vi "UDP LA SEND.vi"() -> ()   [LabVIEW 2017]
uses:
  Global 1.vi
panel:
  in  "upper limit":dbl
  in  "lower limit":dbl
  in  "*/":dbl
  in  "+-":i32
  in  "*/compensate":bool
  in  "+-compensate":bool
  out "LA position":i32
  out "decimal integer string":string
  in  "number 2":dbl(knob) scale=-500.0..500.0
  in  "Stop":bool
  # "100def"
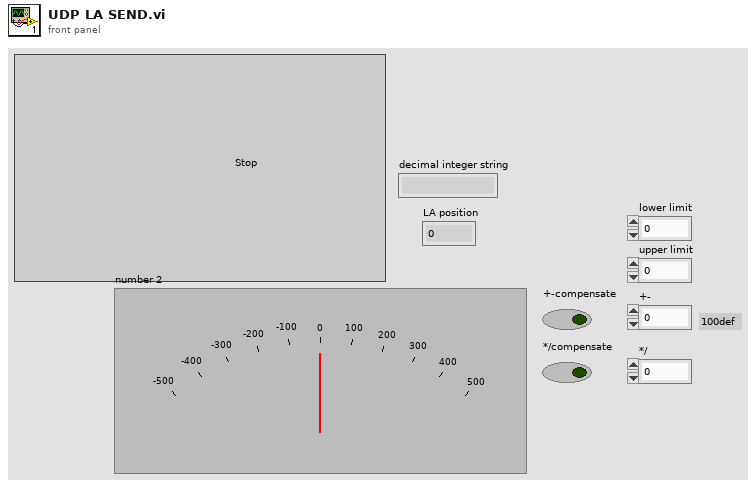
[diagram p1: front panel]
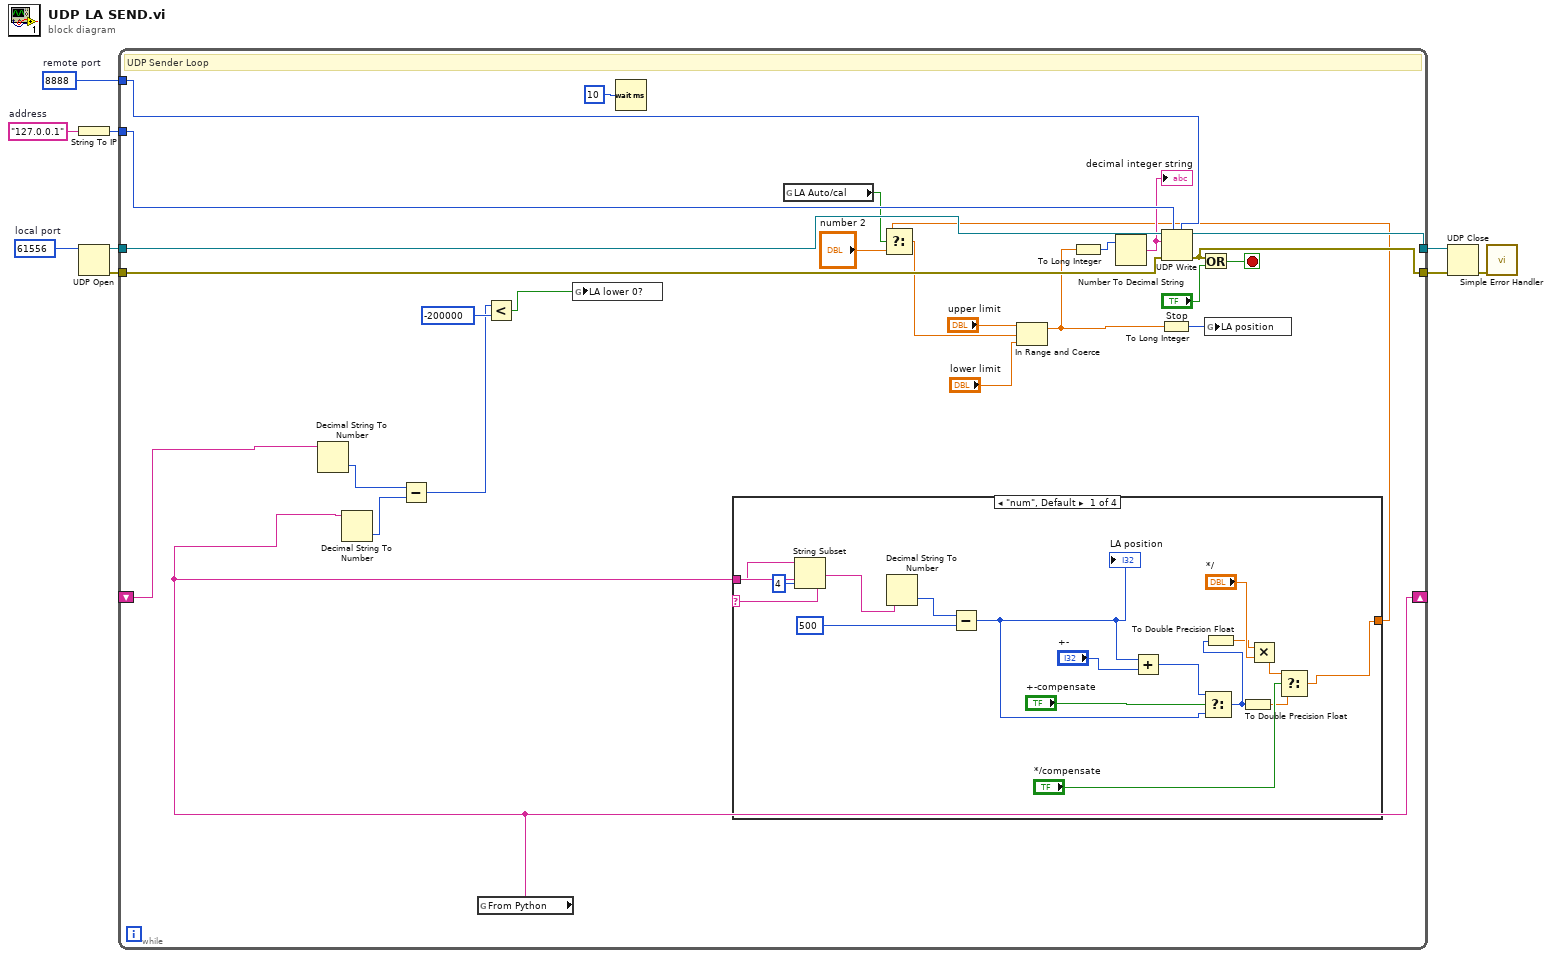
[diagram p0: block diagram]
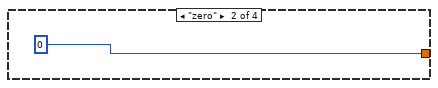
[diagram p2: hidden frame]
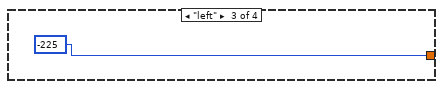
[diagram p3: hidden frame]
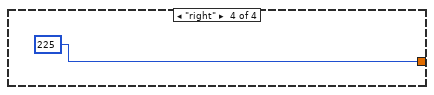
[diagram p4: hidden frame]
diagram:
  w1 = u16 8888  # remote port
  w2 = u16 61556  # local port
  w7 = "127.0.0.1"  # address
  n1 = String To IP(1:w7) -> (0:w5:u32)
  n2 = UDP Open(11:w2) -> (port=w4:refnum<k16>, 0:w3:errorcluster)  [unwired: 4 in, 1 out]
  n3 = while {
    tunnel: [w30] -> w8
    tunnel: w4 -> [w35]
    tunnel: w3 -> [w34]
    tunnel: [w31] -> w9
    tunnel: w5 -> [w29]
    tunnel: w1 -> [w27]
    shift-right: [w16] -> _
    shift-left: _ -> [w17]
    stop <- w33 stop-if-true
    # "UDP Sender Loop"
    n4 = Decimal String To Number(string=w17) -> (number=w22:i32)  [unwired: 2 in, 1 out]
    n5 = global read "Global 1.vi" "From Python"() -> (w16:string)
    n6 = Decimal String To Number(string=w16) -> (number=w18:i32)  [unwired: 2 in, 1 out]
    n7 = Subtract(x=w22, y=w18) -> (x-y=w19:i32)
    n8 = Less?(x=w19, y=-200000) -> (x < y?=w20:bool)
    n9 = global write "Global 1.vi" "LA lower 0?"(w20) -> ()
    n10 = Wait (ms)(milliseconds to wait=u32 10) -> ()  [unwired: 1 out]
    n11 = case shown="\"num\", Default" w16 {
      tunnel: w16 -> [w51 _ _ _]
      tunnel: [w40 0 -225 225] -> w23
      frame "num", Default {
        n12 = String Subset(string=w51, length (rest)=4 ("length (rest)")) -> (substring=w49:string)  [unwired: 1 in]
        n13 = Decimal String To Number(string=w49) -> (number=w48:i32)  [unwired: 2 in, 1 out]
        n14 = Subtract(x=w48, y=500) -> (x-y=w39:i32)
        "LA position" <- w39
        n15 = Add(x=w39, y="+-") -> (x+y=w44:i32)
        n16 = Select(t=w44, s="+-compensate", f=w39) -> (s? t:f=w37:i32)
        n17 = To Double Precision Float(number=w37) -> (double precision float=w38:dbl)
        n18 = To Double Precision Float(number=w37) -> (double precision float=w36:dbl)
        n19 = Multiply(x=w38, y="*/") -> (x*y=w41:dbl)
        n20 = Select(t=w41, s="*/compensate", f=w36) -> (s? t:f=w40:dbl)
      }
      frame "zero" {
      }
      frame "left" {
      }
      frame "right" {
      }
    }
    n21 = global read "Global 1.vi" "LA Auto/cal"() -> (w24:bool)
    n22 = Select(t=w23, s=w24, f="number 2") -> (s? t:f=w12:dbl)
    n23 = In Range and Coerce(upper limit="upper limit", x=w12, lower limit="lower limit") -> (coerced(x)=w10:dbl)  [unwired: 1 out]
    n24 = To Long Integer(number=w10) -> (32bit integer=w11:i32)
    n25 = Number To Decimal String(number=w11) -> (decimal integer string=w28:string)  [unwired: 1 in]
    "decimal integer string" <- w28
    n26 = To Long Integer(number=w10) -> (32bit integer=w13:i32)
    n27 = UDP Write(address=w29, port or service name=w27, connection ID=w35, data in=w28, 8:w34) -> (error out=w30:errorcluster, 3:w31:refnum<k16>)  [unwired: 1 in]
    n28 = Or(x=w30, y="Stop") -> (x .or. y?=w33:bool)
    n29 = global write "Global 1.vi" "LA position"(w13) -> ()
  }
  n30 = UDP Close(connection ID=w9, 8:w8) -> (error out=w6:errorcluster)  [unwired: 1 out]
  n31 = call <vilib>:"Simple Error Handler.vi"("error in (no error)"=w6) -> ()  [unwired: 4 in, 5 out]
